vi "Register for Actor Core Events.vi"(7 "Use Label Text (F=Use Caption)":bool, 8 "error in (no error)":errorcluster, 9 "Controls to Exclude":refnum<vi>[](array[refnum]), 10 "VI Refnum (Calling VI)":refnum<vi>, 11 "Actor Enqueuer":refnum<class "Message Enqueuer.lvclass">) -> (0 "error out":errorcluster, 3 "ActorAutoRegistration Out":refnum<class "ActorAutoRegistration.lvclass">)   [LabVIEW 2015, in "ActorEvents.lvlib" / "ActorAutoRegistration.lvclass"]
doc: "<License>\nCopyright © 2017 Composed Systems, LLC | All rights reserved\nwww.composed.io\n\nAuthor: Ethan Stern <ethan.stern@composed.io>\n\nThis software is provided \"AS IS\" WITHOUT WARRANTIES, either express or implied, AND IS FOR EDUCATIONAL PURPOSES ONLY.\n</License>"
uses:
  ActorAutoRegistration.lvclass
  <vilib>/ActorFramework/Message Enqueuer/Message Enqueuer.lvclass
  ActorAutoRegistration.lvclass/ActorAutoRegistration.ctl
  AutoRegistration/AutoRegistration.lvclass
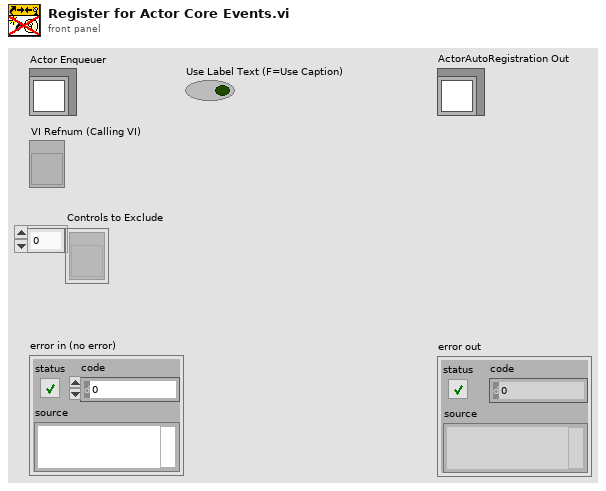
[diagram p1: front panel]
types:
  T1 = typedef "AutoRegistration.lvlib/AutoRegistration.lvclass/Auto-Event Registration Refnum.ctl" = refnum<event-registration>
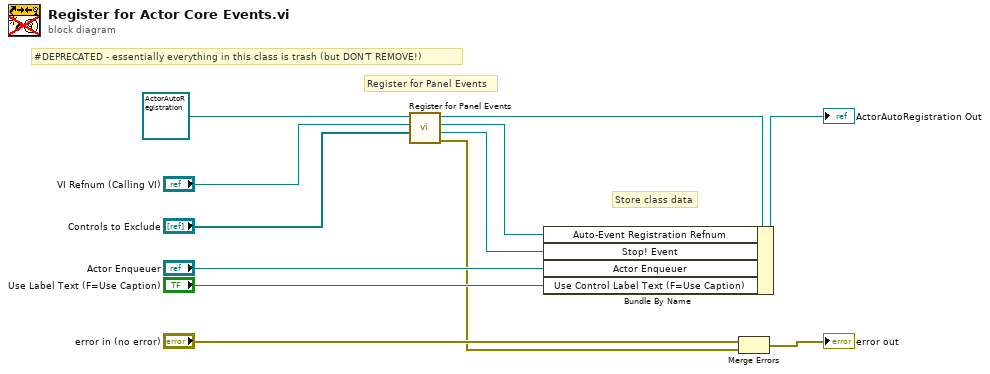
[diagram p0: block diagram]
diagram:
  # "#DEPRECATED - essentially everything in this class is trash (but DON'T REMOVE!)"
  # "Store class data"
  # "Register for Panel Events"
  n1 = call "Register for Panel Events.vi"("Controls to Exclude"="Controls to Exclude", "VI Refnum (Calling VI)"="VI Refnum (Calling VI)", "AbstractAutoRegistration In"=refnum<class "ActorAutoRegistration.lvclass"> refnum ("AbstractAutoRegistration in")) -> ("error out"=w2:errorcluster, "Stop! Event"=w6:refnum<user-event>, "Auto-Event Registration Refnum"=w7:T1, "AbstractAutoRegistration out"=w8:refnum<class "ActorAutoRegistration.lvclass">)  [unwired: 5 in]
  n2 = Bundle By Name(cluster=w8, "Auto-Event Registration Refnum"=w7, "Stop! Event"=w6, "Actor Enqueuer"="Actor Enqueuer", "Use Control Label Text (F=Use Caption)"="Use Label Text (F=Use Caption)") -> (→"ActorAutoRegistration Out":refnum<class "ActorAutoRegistration.lvclass">)
  n3 = Merge Errors("error in (no error)", w2) -> (→"error out":errorcluster)
